vi "user input.vi"(8 "error in":errorcluster) -> (0 "error out":errorcluster, 3 "Inputs from system":T1)   [LabVIEW 2017, in "Central Error Handler runtime.lvclass"]
uses:
  Central Error Handler runtime.lvclass
  input user data.ctl
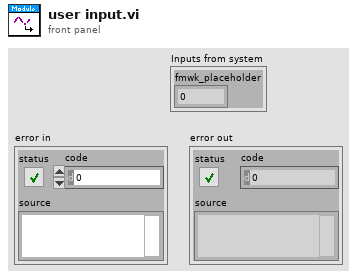
[diagram p1: front panel]
types:
  T1 = typedef "Central Error Handler runtime.lvclass/input user data.ctl" = cluster{"fmwk_placeholder":i32}
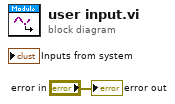
[diagram p0: block diagram]
diagram:
  "error out" <- "error in"
